vi "Read Str.vi"(8 "Error In":errorcluster) -> (0 "Error Out":errorcluster)   [LabVIEW 2017, in "Tests.lvlib" / "Reader.lvlib"]
uses:
  Reader.lvlib
  src/LabPack/Public/Reader/Reader.lvclass/Reader.ctl
  src/LabPack/Public/Reader/Public/Raw/Read Bytes.vi
  src/LabPack/Public/Reader/Private/Read Bytes by Value.vi
  src/LabPack/Public/Reader/Private/Handle Error.vi
  src/LabPack/Public/Reader/Public/Status/Read Status.vi
  src/LabPack/Public/Reader/Public/Status/Read Status Message.vi
  src/LabPack/Public/Reader/Public/Status/Read Is Error.vi
  src/LabPack/Public/Reader/Public/String/Begin Str.vi
  src/LabPack/Public/Reader/Private/Begin Str by Value.vi
  src/LabPack/Public/Utility/Status Code.vi
  <vilib>/Utility/error.llb/Error Cluster From Error Code.vi
  src/LabPack/Public/Reader/Public/String/End Str.vi
  src/LabPack/Public/Reader/Private/End Str by Value.vi
  <vilib>/addons/_JKI Toolkits/Caraya/classes/Test/Test.lvclass
  <vilib>/addons/_JKI Toolkits/Caraya/classes/Assert/Assert.lvclass
  src/LabPack/Public/Reader/Reader.lvclass
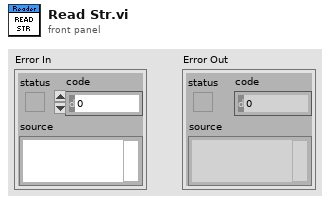
[diagram p1: front panel]
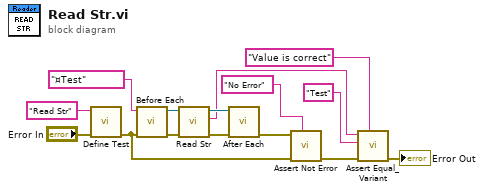
[diagram p0: block diagram]
diagram:
  n1 = call <vilib>:"Define Test.vi"("error in (no error)"="Error In", "Label (VI Title)"="Read Str") -> ("error out"=w12:errorcluster)  [unwired: 9 in]
  n2 = call "Before Each.vi"("Error In"=w12, "Data"="¤Test") -> ("Error Out"=w7:errorcluster, "Reader"=w8:refnum<class "Reader.lvclass">)  [unwired: 8 in]
  n3 = call "Read Str.vi"("Error In"=w7, "Reader In"=w8) -> ("Error Out"=w10:errorcluster, "Value"=w2:string, "Reader Out"=w9:refnum<class "Reader.lvclass">)  [unwired: 7 in]
  n4 = call "After Each.vi"("Error In"=w10, "Reader In"=w9) -> ("Error Out"=w13:errorcluster)  [unwired: 9 in]
  n5 = call <vilib>:"Assert Not Error.vi"("Label"="No Error", "error in (no error)"=w12, "Not Error?"=w13) -> ("error out"=w11:errorcluster)  [unwired: 8 in]
  n6 = call <vilib>:"Assert Equal_Variant.vi"("Label"="Value is correct", "error in (no error)"=w11, "Y"="Test" ("Value"), "X"=w2) -> ("error out"=→"Error Out":errorcluster)  [unwired: 7 in]
